vi "AM - Modulation & De-Modulation.vi"() -> ()   [LabVIEW 2020]
uses:
  <vilib>/express/express analysis/Spectral/Block/exnSpectralBlock spectral measurements peak poly.vi
  <vilib>/express/express analysis/Spectral/Block/exnSpectralBlock spectral measurements peak DDT.vi
  <vilib>/express/express analysis/Spectral/XNode/ExpressSpectralMeasurementsBlockNode.xnode
panel:
  in  "Select Demodulation Method":T1(radio)=enum."synchrounes"
  in  "Select signal":T2(radio)=enum."sine"
  out "time domain":dynamicdata(graph)
  out "spectrum":dynamicdata(graph)
  in  "carrier Phase":dbl=90.0 caption="Phase"
  in  "carrier Offset":dbl caption="Offset"
  in  "carrier Frequency":dbl=100.0 caption="Frequency"
  in  "carrier Amplitude":dbl=1.0 caption="Amplitude"
  out "Frequency domain":dynamicdata(graph)
  out "time domain":dynamicdata(graph)
  in  "DC (A)":dbl
  in  "stop":bool
  in  "Phase":dbl
  in  "Offset":dbl
  in  "Frequency":dbl=10.1
  in  "Amplitude":dbl=1.0
  # "1st button : sine signal\n2nd button: square signal\n3rd button : sawtooth signal \n4th button : trianle signal"
  # "1st button : synchrounes\n2nd button: envelope detector\n3rd button : rectifier detector"
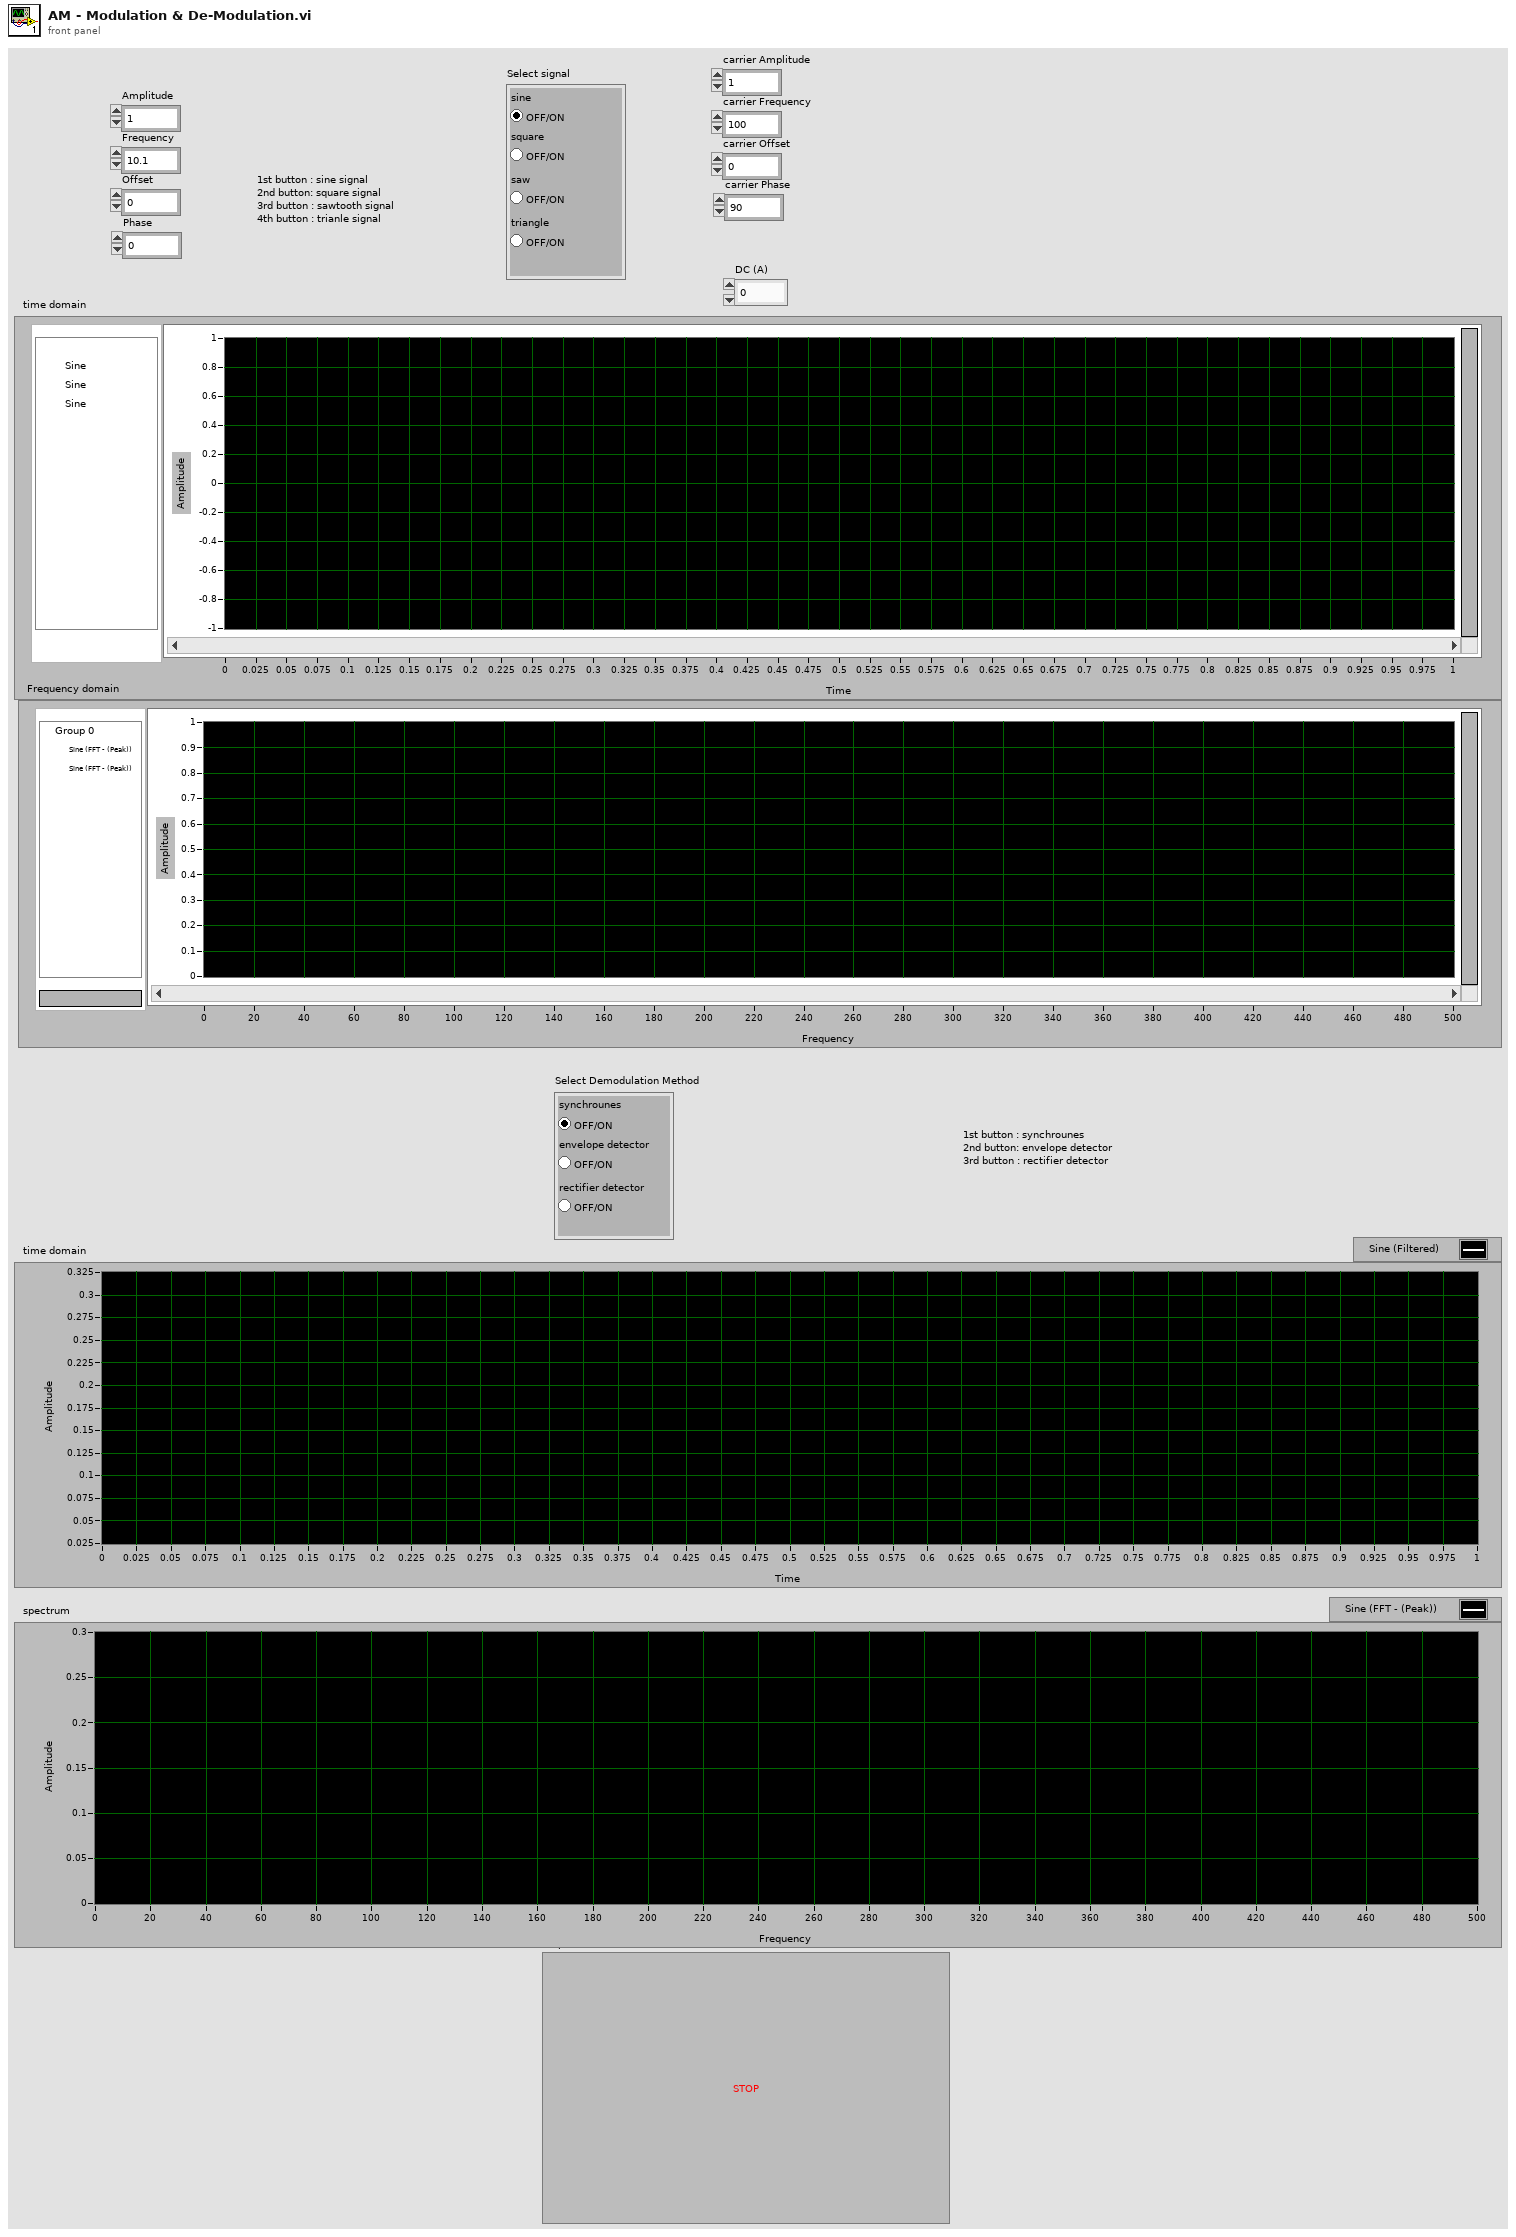
[diagram p1: front panel]
types:
  T1 = enum32{"No Selection", "synchrounes", "envelope detector", "rectifier detector"}
  T2 = enum32{"No Selection", "sine", "square", "saw", "triangle"}
  T3 = cluster{"averaging mode":u16, "weighting mode":u16, "number of averages":u32}
  T4 = cluster{"dB On (F)":bool, "unwrap phase (F)":bool, "convert to degree (F)":bool}
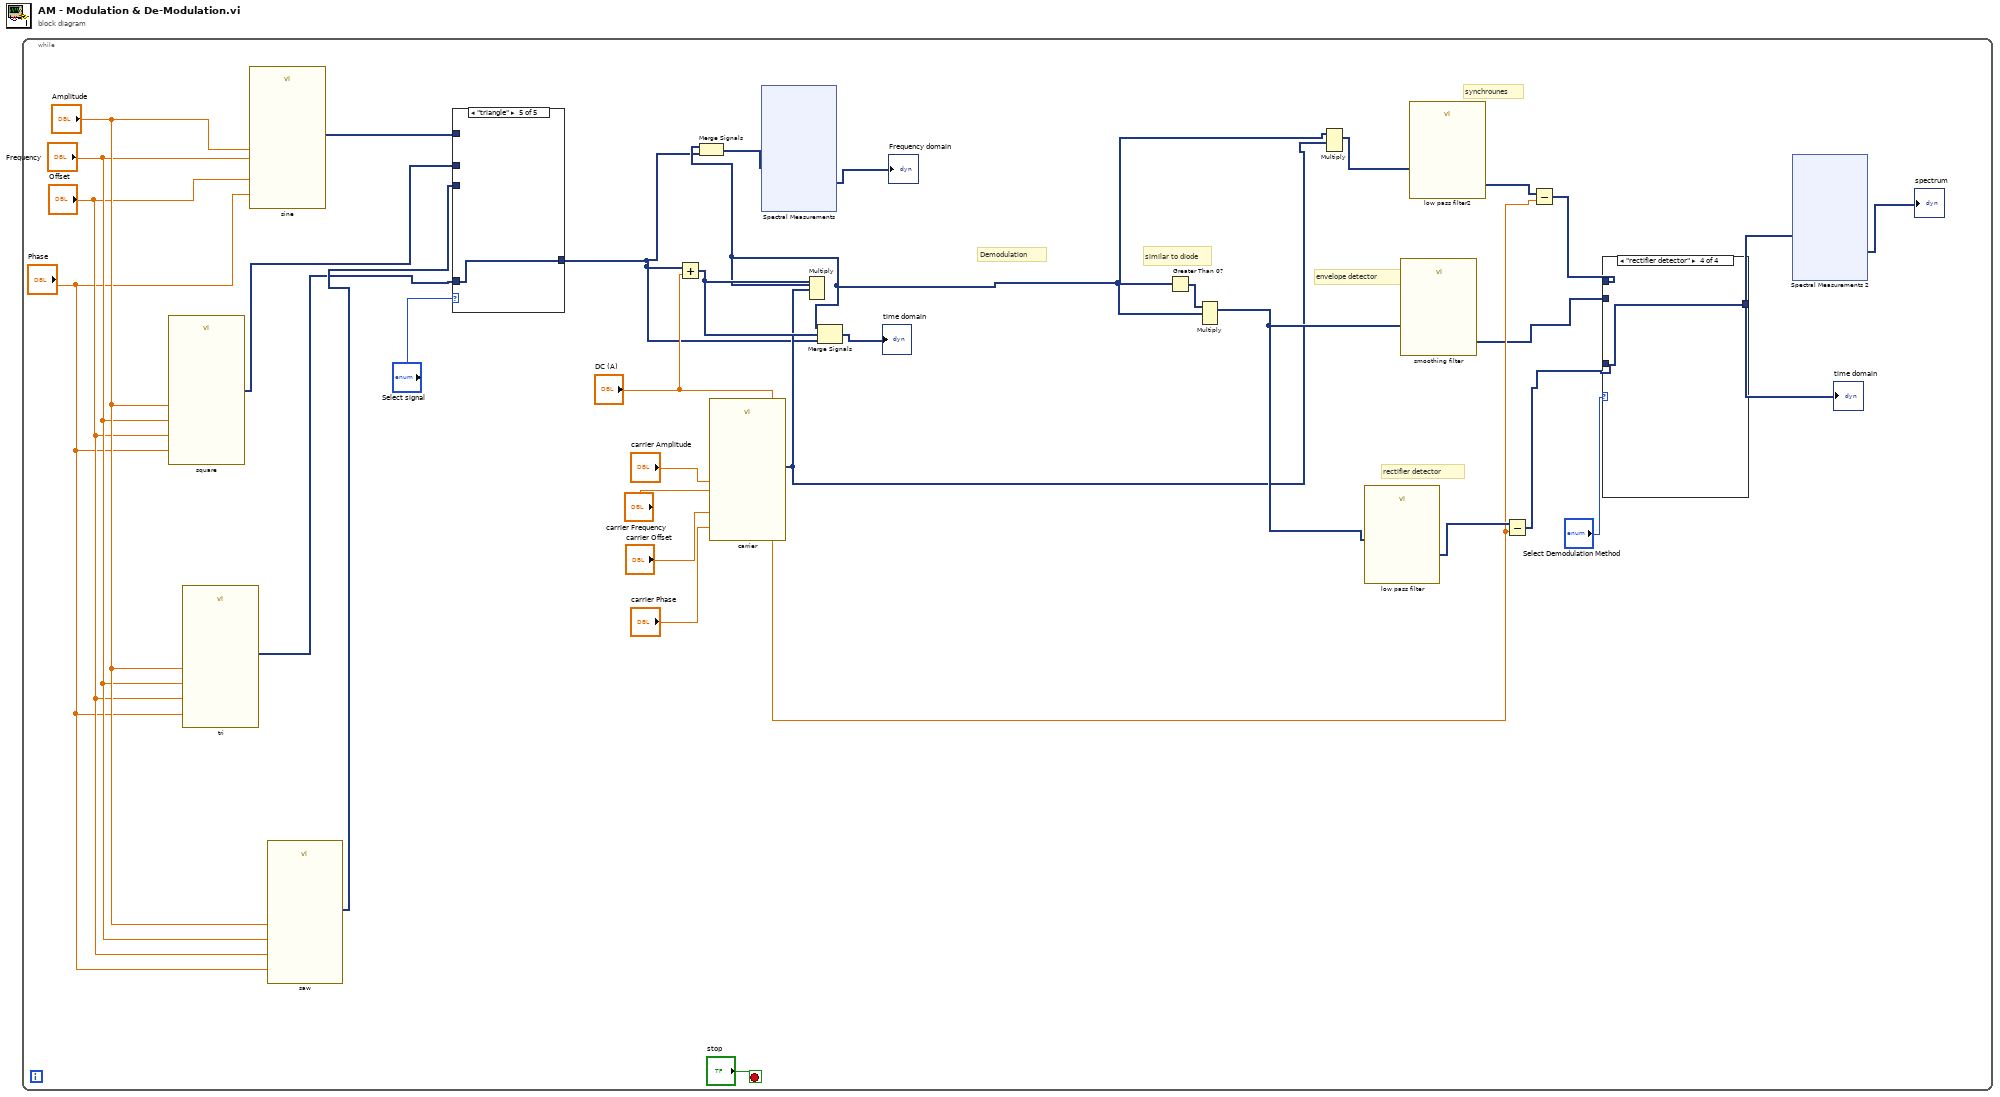
[diagram p0: block diagram]
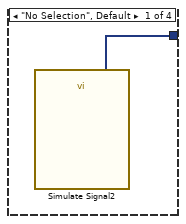
[diagram p2: hidden frame]
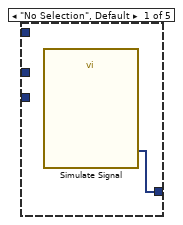
[diagram p5: hidden frame]
diagram:
  n1 = while {
    stop <- "stop" stop-if-true
    # "rectifier detector"
    # "envelope detector"
    # "synchrounes"
    # "Demodulation"
    # "similar to diode"
    n2 = call "square"("Offset"="Offset", "Frequency"="Frequency", "Amplitude"="Amplitude", "Phase"="Phase") -> ("Square"=w9:dynamicdata)  [unwired: 10 in, 1 out]
    n3 = call "tri"("Offset"="Offset", "Frequency"="Frequency", "Amplitude"="Amplitude", "Phase"="Phase") -> ("Triangle"=w7:dynamicdata)  [unwired: 10 in, 1 out]
    n4 = call "sine"("Offset"="Offset", "Frequency"="Frequency", "Amplitude"="Amplitude", "Phase"="Phase") -> ("Sine"=w10:dynamicdata)  [unwired: 10 in, 1 out]
    n5 = call "saw"("Offset"="Offset", "Frequency"="Frequency", "Amplitude"="Amplitude", "Phase"="Phase") -> ("Sawtooth"=w8:dynamicdata)  [unwired: 10 in, 1 out]
    n6 = case shown="\"triangle\"" "Select signal" {
      tunnel: [w38 w39 w40 w41 w42] -> w11
      tunnel: w10 -> [_ w39 _ _ _]
      tunnel: w9 -> [_ _ w40 _ _]
      tunnel: w8 -> [_ _ _ w41 _]
      tunnel: w7 -> [_ _ _ _ w42]
      frame "No Selection", Default {
        n7 = call "Simulate Signal"() -> ("Sine"=w38:dynamicdata)  [unwired: 14 in, 1 out]
      }
      frame "sine" {
      }
      frame "square" {
      }
      frame "saw" {
      }
      frame "triangle" {
      }
    }
    n8 = Add(x=w11, y="DC (A)") -> (x+y=w29:dynamicdata)
    n9 = call "carrier"("Offset"="carrier Offset", "Frequency"="carrier Frequency", "Amplitude"="carrier Amplitude", "Phase"="carrier Phase") -> ("Sine"=w25:dynamicdata)  [unwired: 10 in, 1 out]
    n10 = Multiply(1:w25, 2:w29) -> (0:w23:dynamicdata)  [unwired: 1 in, 1 out]
    n11 = Merge Signals(w23, w11) -> (w31:dynamicdata)
    n12 = xnode "Spectral Measurements"("Signals"=w31) -> ("FFT - (Peak)"=→"Frequency domain":dynamicdata)  [unwired: 1 in, 2 out]
    n13 = Merge Signals(w23, w29, w11) -> (→"time domain":dynamicdata)
    n14 = Greater Than 0?(x=w23) -> (x > 0?=w28:dynamicdata)
    n15 = Multiply(1:w23, 2:w28) -> (0:w27:dynamicdata)  [unwired: 1 in, 1 out]
    n16 = Multiply(1:w25, 2:w23) -> (0:w24:dynamicdata)  [unwired: 1 in, 1 out]
    n17 = call "low pass filter"("Signal"=w27) -> ("Filtered Signal"=w26:dynamicdata)  [unwired: 9 in, 1 out]
    n18 = call "smoothing filter"("Signal"=w27) -> ("Filtered Signal"=w4:dynamicdata)  [unwired: 9 in, 1 out]
    n19 = call "low pass filter2"("Signal"=w24) -> ("Filtered Signal"=w16:dynamicdata)  [unwired: 9 in, 1 out]
    n20 = Subtract(x=w26, y="DC (A)") -> (x-y=w3:dynamicdata)
    n21 = Subtract(x=w16, y="DC (A)") -> (x-y=w5:dynamicdata)
    n22 = case shown="\"rectifier detector\"" "Select Demodulation Method" {
      tunnel: w5 -> [_ w35 _ _]
      tunnel: w4 -> [_ _ w36 _]
      tunnel: w3 -> [_ _ _ w37]
      tunnel: [w34 w35 w36 w37] -> w1
      frame "No Selection", Default {
        n23 = call "Simulate Signal2"() -> ("Sine"=w34:dynamicdata)  [unwired: 14 in, 1 out]
      }
      frame "synchrounes" {
      }
      frame "envelope detector" {
      }
      frame "rectifier detector" {
      }
    }
    "time domain" <- w1
    n24 = xnode "Spectral Measurements 2"("Signals"=w1) -> ("FFT - (Peak)"=→"spectrum":dynamicdata)  [unwired: 1 in, 2 out]
  }
